vi "Add Target 2 Command Data.vi"(6 "Combined":bool, 9 "LBCB 2 Command Data In":T1, 10 "LBCB 1 Command Data In":T1, 11 "Target":T2) -> (1 "LBCB 2 Command Data Out":T1, 2 "LBCB 1 Command Data Out":T1)   [LabVIEW 2009]
uses:
  MixedMode/Messages/Target.ctl
  Data Access Objects/Metadata/LBCB Number.ctl
  MixedMode/Target Data.ctl
  Global Data/Transactions/Dataset Transaction Id.ctl
  Global Data/Transactions/Dataset Source.ctl
  Global Data/Transactions/Dataset Type.ctl
  Apps/Yes No Button.ctl
  Data Access Objects/Metadata/DAO Actions.ctl
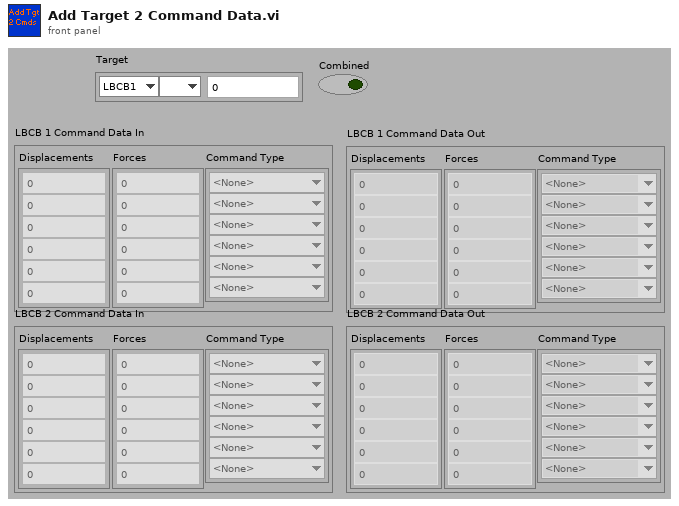
[diagram p1: front panel]
types:
  T1 = typedef "Target Data.ctl" = cluster{"Displacements":dbl[], "Command Type":enum16{"<None>", "Displacement", "Force"}[], "Forces":dbl[]}
  T2 = typedef "Target.ctl" = cluster{"LBCB Number":T3, "DOF Vectors":enum16{" ", "Dx", "Dy", "Dz", "Rx", "Ry", "Rz", "Fx", "Fy", "Fz", "Mx", "My", "Mz"}, "Amount":dbl}
  T3 = typedef "LBCB Number.ctl" = enum16{"LBCB1", "LBCB2"}
  T4 = typedef "DAO Actions.ctl" = enum16{"Init", "Get", "Set"}
  T5 = typedef "Dataset Type.ctl" = enum16{"LVDT", "Load Cell", "Actuator Command", "Servo Error", "Displacement Command", "Displacement", "Force"}
  T6 = typedef "Dataset Transaction Id.ctl" = cluster{"Dataset Source":T7, "Dataset Type":T5, "Hold":T8, "Volts":T8, "Tag":string}
  T7 = typedef "Dataset Source.ctl" = enum16{"LBCB 1", "LBCB 2", "Combined", "External Sensors"}
  T8 = typedef "Yes No Button.ctl" = bool
  T9 = enum16{" ", "Dx", "Dy", "Dz", "Rx", "Ry", "Rz", "Fx", "Fy", "Fz", "Mx", "My", "Mz"}
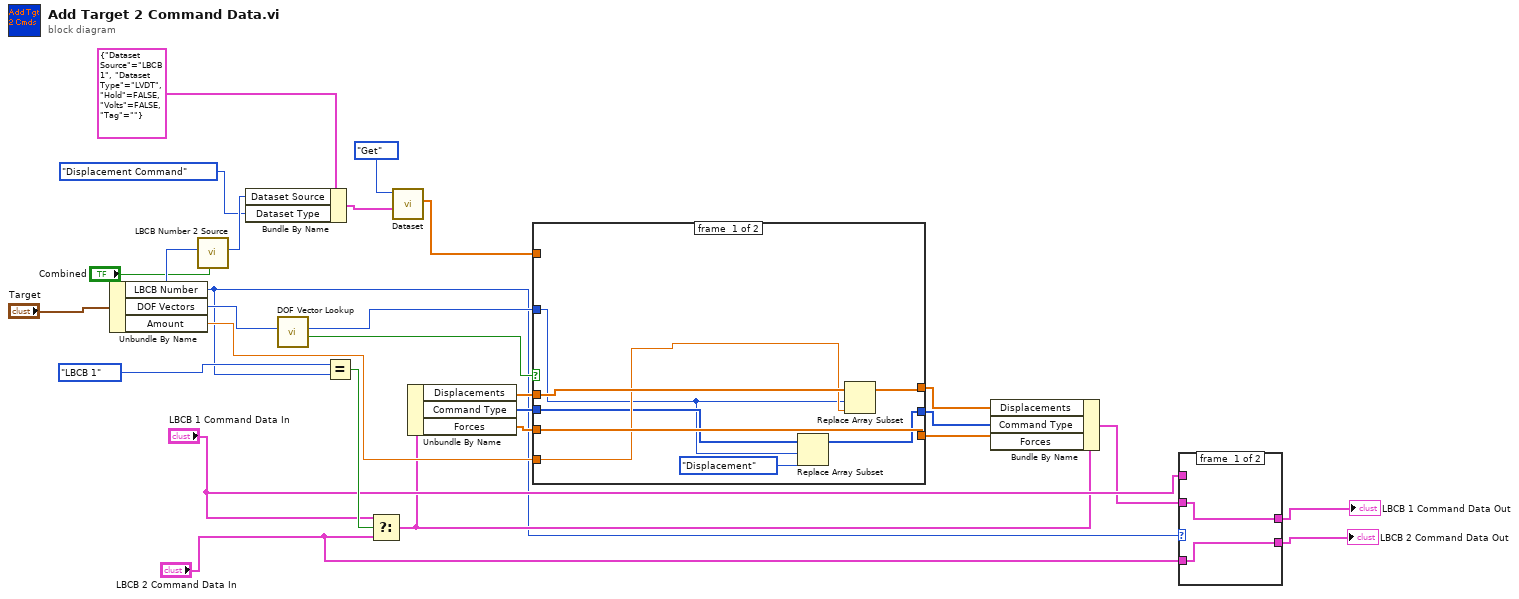
[diagram p0: block diagram]
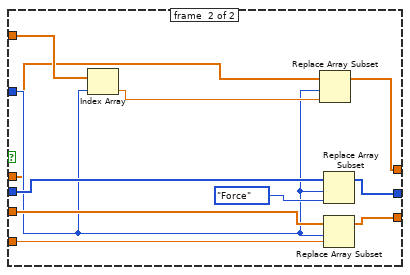
[diagram p2: hidden frame]
diagram:
  n1 = Unbundle By Name("Target") -> ("LBCB Number"=w5:T3, "DOF Vectors"=w26:T9, "Amount"=w14:dbl)
  n2 = call "LBCB Number 2 Source.vi"("Combined"="Combined", "LBCB Number"=w5) -> ("Dataset Source"=w7:T7)  [unwired: 9 in]
  n3 = Bundle By Name(cluster=T6 {"Dataset Source"=enum."LBCB 1", "Dataset Type"=enum."LVDT", "Hold"=FALSE, "Volts"=FALSE, "Tag"=""} ("Dataset Trans Id"), "Dataset Source"=w7, "Dataset Type"=Dataset_Type."Displacement Command" ("f")) -> (w8:T6)
  n4 = call "DOF Vector Lookup.vi"("DOF Vectors"=w26) -> ("IsForce"=w19:bool, "Index"=w15:u32)  [unwired: 9 out]
  n5 = Equal?(x=enum16{"LBCB 1", "LBCB 2"}."LBCB 1", y=w5) -> (x = y?=w25:bool)
  n6 = Select(t="LBCB 1 Command Data In", s=w25, f="LBCB 2 Command Data In") -> (s? t:f=w13:T1)
  n7 = call "Dataset.vi"("Dataset Trans Id"=w8, "DAO Actions"=DAO_Actions."Get") -> ("Data Out"=w2:dbl[])  [unwired: 8 in, 1 out]
  n8 = Unbundle By Name(w13) -> ("Displacements"=w18:dbl[], "Command Type"=w16:enum16{"<None>", "Displacement", "Force"}[], "Forces"=w17:dbl[])
  n9 = case shown="False" w19 {
    tunnel: w18 -> [w35 w37]
    tunnel: w17 -> [w33 w45]
    tunnel: w16 -> [w31 w46]
    tunnel: w15 -> [w30 w38]
    tunnel: w14 -> [w32 w42]
    tunnel: [w34 w36] -> w12
    tunnel: [w28 w44] -> w11
    tunnel: [w33 w43] -> w10
    tunnel: w2 -> [_ w40]
    frame #0 {
      n10 = Replace Array Subset(array=w31, new element=enum16{"<None>", "Displacement", "Force"}."Displacement" ("Enum"), index=w30) -> (w28:enum16{"<None>", "Displacement", "Force"}[])
      n11 = Replace Array Subset(array=w35, new element=w32, index=w30) -> (w34:dbl[])
    }
    frame #1 {
      n12 = Index Array(array=w40, index=w38) -> (element=w39:dbl)
      n13 = Replace Array Subset(array=w37, new element=w39, index=w38) -> (w36:dbl[])
      n14 = Replace Array Subset(array=w46, new element=enum16{"<None>", "Displacement", "Force"}."Force" ("Enum"), index=w38) -> (w44:enum16{"<None>", "Displacement", "Force"}[])
      n15 = Replace Array Subset(array=w45, new element=w42, index=w38) -> (w43:dbl[])
    }
  }
  n16 = Bundle By Name(cluster=w13, "Displacements"=w12, "Command Type"=w11, "Forces"=w10) -> (w20:T1)
  n17 = case shown="\"LBCB2\"" w5 {
    tunnel: w20 -> [w48 w49]
    tunnel: "LBCB 1 Command Data In" -> [_ w50]
    tunnel: "LBCB 2 Command Data In" -> [w47 _]
    tunnel: [w48 w50] -> w22
    tunnel: [w47 w49] -> w21
    frame #0 {
    }
    frame #1 {
    }
  }
  "LBCB 1 Command Data Out" <- w22
  "LBCB 2 Command Data Out" <- w21
